vi "FindRobotByID.vi"(8 "error in (no error)":errorcluster, 9 "id":i32, 10 "RobotRef":refnum<class "Robot.lvclass">[](array[class]), 11 "Utilities in":refnum<class "Utilities.lvclass">) -> (0 "error out":errorcluster, 1 "index":i32, 2 "Robot":refnum<class "Robot.lvclass">, 3 "Utilities out":refnum<class "Utilities.lvclass">)   [LabVIEW 2023, in "Utilities.lvclass"]
uses:
  Utilities.lvclass
  Robot_class/Robot.lvclass
  Robot_class/Robot.lvclass/Robot.ctl
  Robot_class/Read id.vi
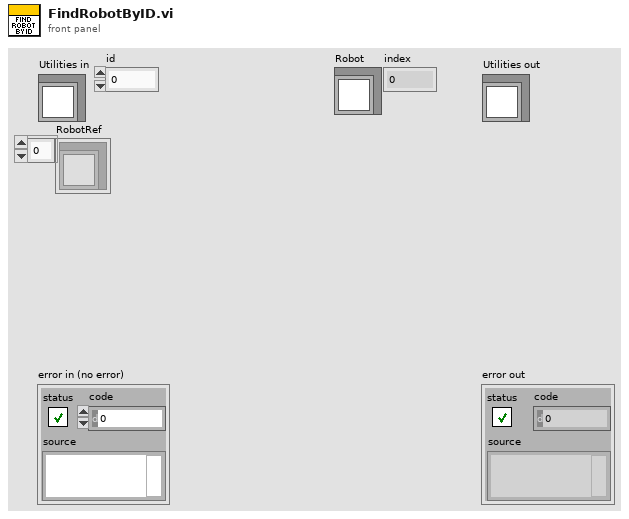
[diagram p1: front panel]
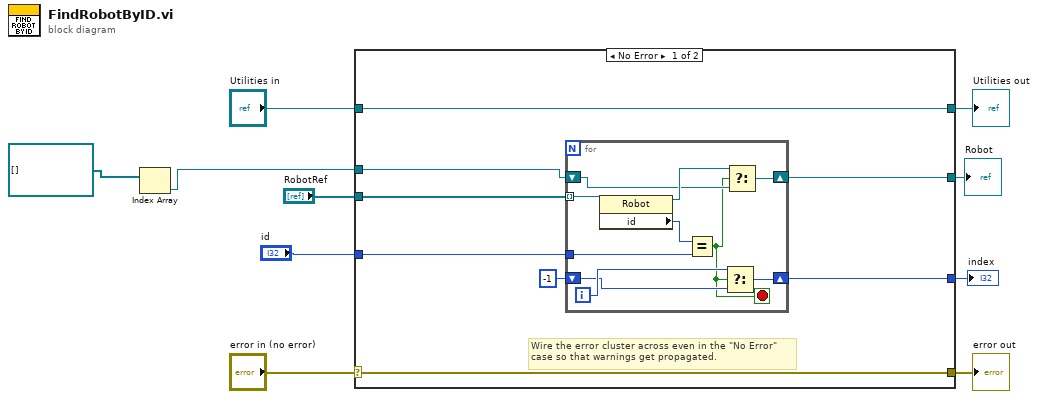
[diagram p0: block diagram]
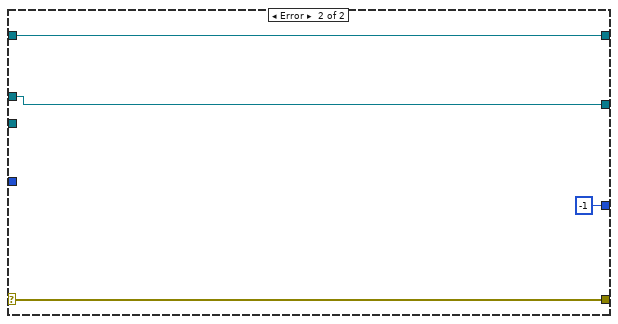
[diagram p2: hidden frame]
diagram:
  n1 = Index Array(array=refnum<class "Robot.lvclass">[] []) -> (element=w1:refnum<class "Robot.lvclass">)  [unwired: 1 in]
  n2 = case shown="No Error" "error in (no error)" {
    selector: "error in (no error)" -> [w17 w32]
    tunnel: [w17 w32] -> w9
    tunnel: [w18 w31] -> w7
    tunnel: "Utilities in" -> [w18 w31]
    tunnel: "RobotRef" -> [w16 _]
    tunnel: "id" -> [w15 _]
    tunnel: [w14 w30] -> w4
    tunnel: w1 -> [w13 w30]
    tunnel: [w11 -1] -> w3
    frame No Error {
      # "Wire the error cluster across even in the \"No Error\"\ncase so that warnings get propagated."
      n3 = for {
        tunnel: w16 -> [w28] mode=indexing
        tunnel: w15 -> [w26]
        shift-right: [w24] -> w14
        shift-left: w13 -> [w23]
        shift-right: [w21] -> w11
        shift-left: -1 -> [w20]
        i -> [w22]
        stop <- w19 stop-if-true
        n4 = property class="Robot"(reference=w28) -> (reference out=w25:refnum<class "Robot.lvclass">, "id"=w27:i32)  [unwired: 1 in, 1 out]
        n5 = Equal?(x=w27, y=w26) -> (x = y?=w19:bool)
        n6 = Select(t=w22, s=w19, f=w20) -> (s? t:f=w21:i32)
        n7 = Select(t=w25, s=w19, f=w23) -> (s? t:f=w24:refnum<class "Robot.lvclass">)
      }
    }
    frame Error {
    }
  }
  "error out" <- w9
  "Utilities out" <- w7
  "Robot" <- w4
  "index" <- w3
